vi "Laser-simples.vi"() -> ()   [LabVIEW 2024]
panel:
  out "String":string
  in  "stop":bool
  in  "on/off":bool
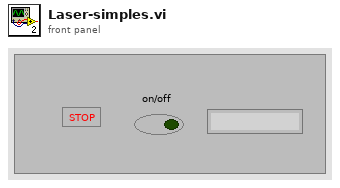
[diagram p1: front panel]
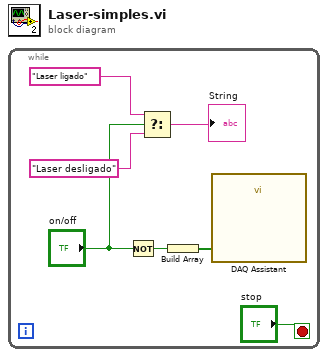
[diagram p0: block diagram]
diagram:
  n1 = while {
    stop <- "stop" stop-if-true
    n2 = Not(x="on/off") -> (.not. x?=w5:bool)
    n3 = Select(t="Laser ligado", s="on/off", f="Laser desligado") -> (s? t:f=→"String":string)
    n4 = Build Array(w5) -> (w6:bool[])
    n5 = call "DAQ Assistant"("data"=w6) -> ()  [unwired: 17 in, 2 out]
  }
